vi "createImage.vi"(8 "error in (no error)":errorcluster, 9 "ImageName":string, 10 "imageString":string, 11 "ImageAnalyser in":refnum<class "ImageAnalyser.lvclass">) -> (0 "error out":errorcluster, 2 "ImageData":T1, 3 "ImageAnalyser out":refnum<class "ImageAnalyser.lvclass">)   [LabVIEW 2009, in "Tools.lvlib" / "Imaging.lvlib" / "ImageAnalyser.lvclass"]
uses:
  ImageAnalyser.lvclass
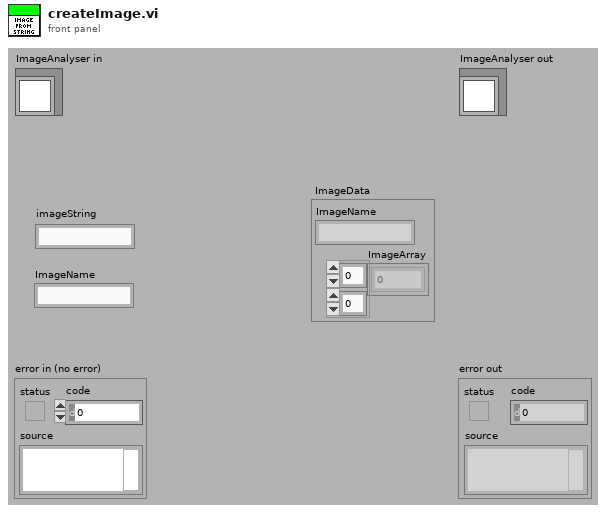
[diagram p1: front panel]
types:
  T1 = cluster{"ImageName":string, "ImageArray":sgl[][]}
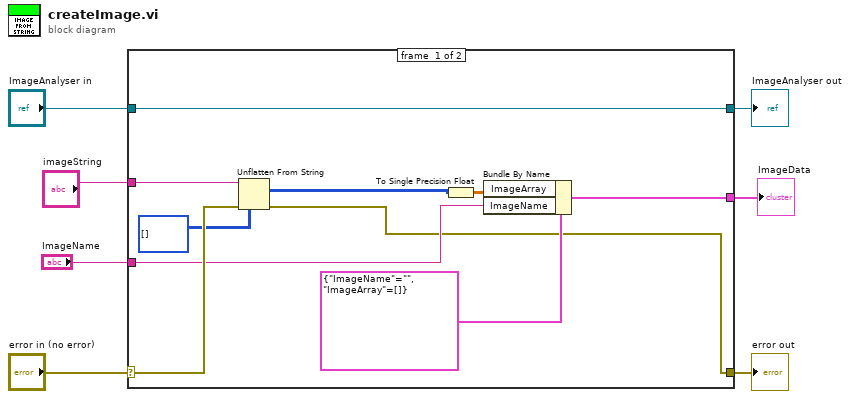
[diagram p0: block diagram]
diagram:
  n1 = case shown="No Error" "error in (no error)" {
    selector: "error in (no error)" -> [w15 w19]
    tunnel: [w10 w19] -> w6
    tunnel: [w17 w18] -> w4
    tunnel: "ImageAnalyser in" -> [w17 w18]
    tunnel: "imageString" -> [w16 _]
    tunnel: "ImageName" -> [w12 _]
    tunnel: [w11 _] -> w1
    frame #0 {
      n2 = Unflatten From String(type=u16[][] [] ("Image data"), binary string=w16, error in (no error)=w15) -> (value=w8:u16[][], error out=w10:errorcluster)  [unwired: 2 in, 1 out]
      n3 = To Single Precision Float(number=w8) -> (single precision float=w9:sgl[][])
      n4 = Bundle By Name(cluster=T1 {"ImageName"="", "ImageArray"=[]}, "ImageArray"=w9, "ImageName"=w12) -> (w11:T1)
    }
    frame #1 {
    }
  }
  "error out" <- w6
  "ImageAnalyser out" <- w4
  "ImageData" <- w1
